vi "slow_control_alpha_07.vi"() -> ()   [LabVIEW 2018]
uses:
  <vilib>/DAQmx/read.llb/DAQmx Read (Analog 1D DBL NChan 1Samp).vi
  <vilib>/DAQmx/create/channels.llb/DAQmx Create Channel (AI-Voltage-Basic).vi
  <vilib>/DAQmx/miscellaneous.llb/DAQmx Fill In Error Info.vi
  <instrlib>/Lake Shore 335/Lake Shore 335.lvlib
  <instrlib>/CAEN PSM/CAEN PSM.lvlib
panel:
  out "Coldhead":dbl
  out "Heater":dbl
  out "Cycle number":i32
  out "TOBA tester":dbl[][](array[numeric])
  in  "Cycles to execute":dbl=5.0 format="%#_13g"
  out "Moving average Det. P":dbl
  in  "N samples":i32=20
  in  "Allows tabs on \nfront panel":T1(tab)
  in  "Heater range":u16(ring) items=["Off", "Low (On)", "Medium", "High"]
  in  "Setpoint (°C)":dbl=-100.0 format="%.1f"
  in  "PID settings":cluster{"P":dbl, "I":dbl, "D":dbl}={"P"=50.0, "I"=20.0, "D"=120.0}
  in  "COM-port LakeShore":refnum<visa-resource-name>
  in  "ID Query":bool=TRUE
  in  "COM-port CAEN 1":refnum<visa-resource-name>
  in  "COM-port CAEN 2":refnum<visa-resource-name>
  in  "Sensor 2 Offset":dbl=1.0 format="%#_13g"
  in  "Sensor 2 Mult. Factor":dbl=25.0 format="%#_13g"
  in  "Sensor 1 Offset":dbl=0.44736 format="%#_13g"
  in  "Sensor 1 Mult. Factor":dbl=25.0 format="%#_13g"
  in  "Sensor 3 Offset":dbl=1.0 format="%#_13g"
  in  "Sensor 3 Mult. Factor":dbl=50.0 format="%#_13g"
  in  "Sensor 4 Offset":dbl=1.0 format="%#_13g"
  in  "Sensor 4 Mult. Factor":dbl=10.0 format="%#_13g"
  out "Heater power (%) 2":cluster{timestamp[], dbl[]}[](graph)
  out "Temp B":dbl
  out "Temp A":dbl
  out "LakeShore readings 2":dbl[](array[numeric])
  in  "Detector Pressure":tag="cDAQ2Mod1/ai0"
  in  "Low Pressure":tag="cDAQ2Mod1/ai1"
  in  "High Pressure":tag="cDAQ2Mod1/ai2"
  in  "Flow Meter":tag="cDAQ2Mod1/ai3"
  out "Corrected P (3x bar, 1x SLPM)":dbl[](array[numeric])
  out "Raw P (Volt)":dbl[](array[numeric]) format="%0.4f"
  in  "Ignore Initialization Errors":bool caption="Ignore init. errors?"
  out "LakeShore status":bool
  out "NI mod1 (P) status":bool
  out "CAEN 1 status":bool
  out "CAEN 2 status":bool
  out "Initialization status":bool
  out "Heater power (%)":cluster{timestamp[], dbl[]}[](graph)
  out "Flow (SLPM)":cluster{timestamp[], dbl[]}[](graph)
  out "Pressure":cluster{timestamp[], dbl[]}[](graph)
  out "Phase Diagram":cluster{"X":dbl, "Y":dbl}[](graph)
  in  "Temp. Channel selector":string(combo)="Average 15 to 20"
  out "Temperature":cluster{timestamp[], dbl[]}[](graph)
  in  "N samples":i32=30
  out "Average Flow (SLPM)":dbl caption="Average Flow (SLPM), of"
  in  "Pause?":bool
  out "Integrated Flow (SL)":dbl
  in  "Reset?":bool
  out "LakeShore readings":dbl[](array[numeric])
  out "Temp. 1":dbl
  out "Temp. 2":dbl
  out "Temp. 3":dbl
  out "Temp. 4":dbl
  out "Temp. 5":dbl
  out "Temp. 6":dbl
  out "Temp. 7":dbl
  out "Temp. 8":dbl
  out "Temp. 9":dbl
  out "Temp. 10":dbl
  out "Temp. 11":dbl
  out "Temp. 12":dbl
  out "Temp. 13":dbl
  out "Temp. 14":dbl
  out "Temp. 15":dbl
  out "Temp. 16":dbl
  out "Temp. 17":dbl
  out "Temp. 18":dbl
  out "Temp. 19":dbl
  out "Temp. 20":dbl
  out "1 to 4":dbl[](array[numeric])
  out "5 to 8":dbl[](array[numeric])
  out "9 to 12":dbl[](array[numeric])
  out "13 to 16":dbl[](array[numeric])
  out "17 to 20":dbl[](array[numeric])
  in  "Temperature Channel selector":string(combo)="Average 15 to 20"
  out "Historical Large Phase Diagram":cluster{dbl[], dbl[]}[](graph)
  out "Large Phase Diagram":cluster{"X":dbl, "Y":dbl}[](graph)
  in  "Temperature Channel selector":string(combo)="Average 15 to 20"
  in  "Set to zero":bool
  out "Bottom gate":dbl(knob) scale=0.0..-3000.0
  out "Top gate":dbl(knob) scale=0.0..3000.0
  in  "Apply Voltage":bool
  in  "VSet (V)":dbl[](array[numeric])
  in  "IMax (uA)":dbl[](array[numeric])
  in  "VMax (V)":dbl[](array[numeric])
  out "Cathode":dbl(knob) scale=0.0..-5000.0
  out "Anode":dbl(knob) scale=0.0..4000.0
  out "PMT 2":dbl(knob) scale=0.0..1000.0
  out "PMT 1":dbl(knob) scale=1.0..1000.0
  out "Vmon (V)":dbl[](array[numeric])
  out "IMon (uA)":dbl[](array[numeric])
  in  "Read V every N cycles":i16=120
  in  "Reset anode":bool
  in  "Kill every Y minutes":i32=10
  in  "Keep off for X seconds":i32=10
  out "?":bool
  out "Killed":bool
  out "Restarted":bool
  out "Anode times":dbl[](array[numeric]) format="%_12f"
  out "Anode times 2":timestamp[](array[timestamp])
  in  "Kill voltage":bool
  in  "stop":bool
  out "Voltages":dbl[](array[numeric])
  out "Started up?":bool
  out "TOBA appended":dbl[][](array[numeric])
  in  "Read T every N cycles":i32=2
  out "Time until next cycle":dbl format="%.3g"
  in  "Time per cycle (s)":i32=2 caption="Time Target (s)"
  # "<- Proof of concept for New/Old T + New P"
  # "PMT 1"
  # "PMT 2"
  # "Anode"
  # "Cathode"
  # "Top gate"
  # "Bottom gate"
  # "Connection settings"
  # "Lakeshore settings"
  # "Pressure sensor settings"
  # "Gain (P) (XX.X)"
  # "Reset (I) (XX.X)"
  # "Rate (D) (X.X%)"
  # "Might need to split up NI-box com port.\nPreferable to task it with measuring T\nand P seperately.\nPerhaps need to set task per single channel."
  # "Heater tests"
  # "Move to Quick Temp tab ^"
  # "Alarm indicators"
  # "CAEN 1"
  # "Data"
  # "PMT 1"
  # "PMT 1"
  # "PMT 2"
  # "PMT 2"
  # "Anode"
  # "Anode"
  # "Cathode"
  # "Cathode"
  # "Top gate"
  # "Top gate"
  # "Bottom gate"
  # "Bottom gate"
  # "Settings"
  # "PMT 1"
  # "PMT 1"
  # "PMT 2"
  # "PMT 2"
  # "Anode"
  # "Anode"
  # "Cathode"
  # "Cathode"
  # "Top gate"
  # "Top gate"
  # "Bottom gate"
  # "Bottom gate"
  # "CAEN 2"
  # "PMT 1"
  # "PMT 2"
  # "Anode"
  # "Cathode"
  # "Needle gauges or other displays go here"
  # "Top gate"
  # "Bottom gate"
  # "Time of last reset"
  # "Time of last reactivation"
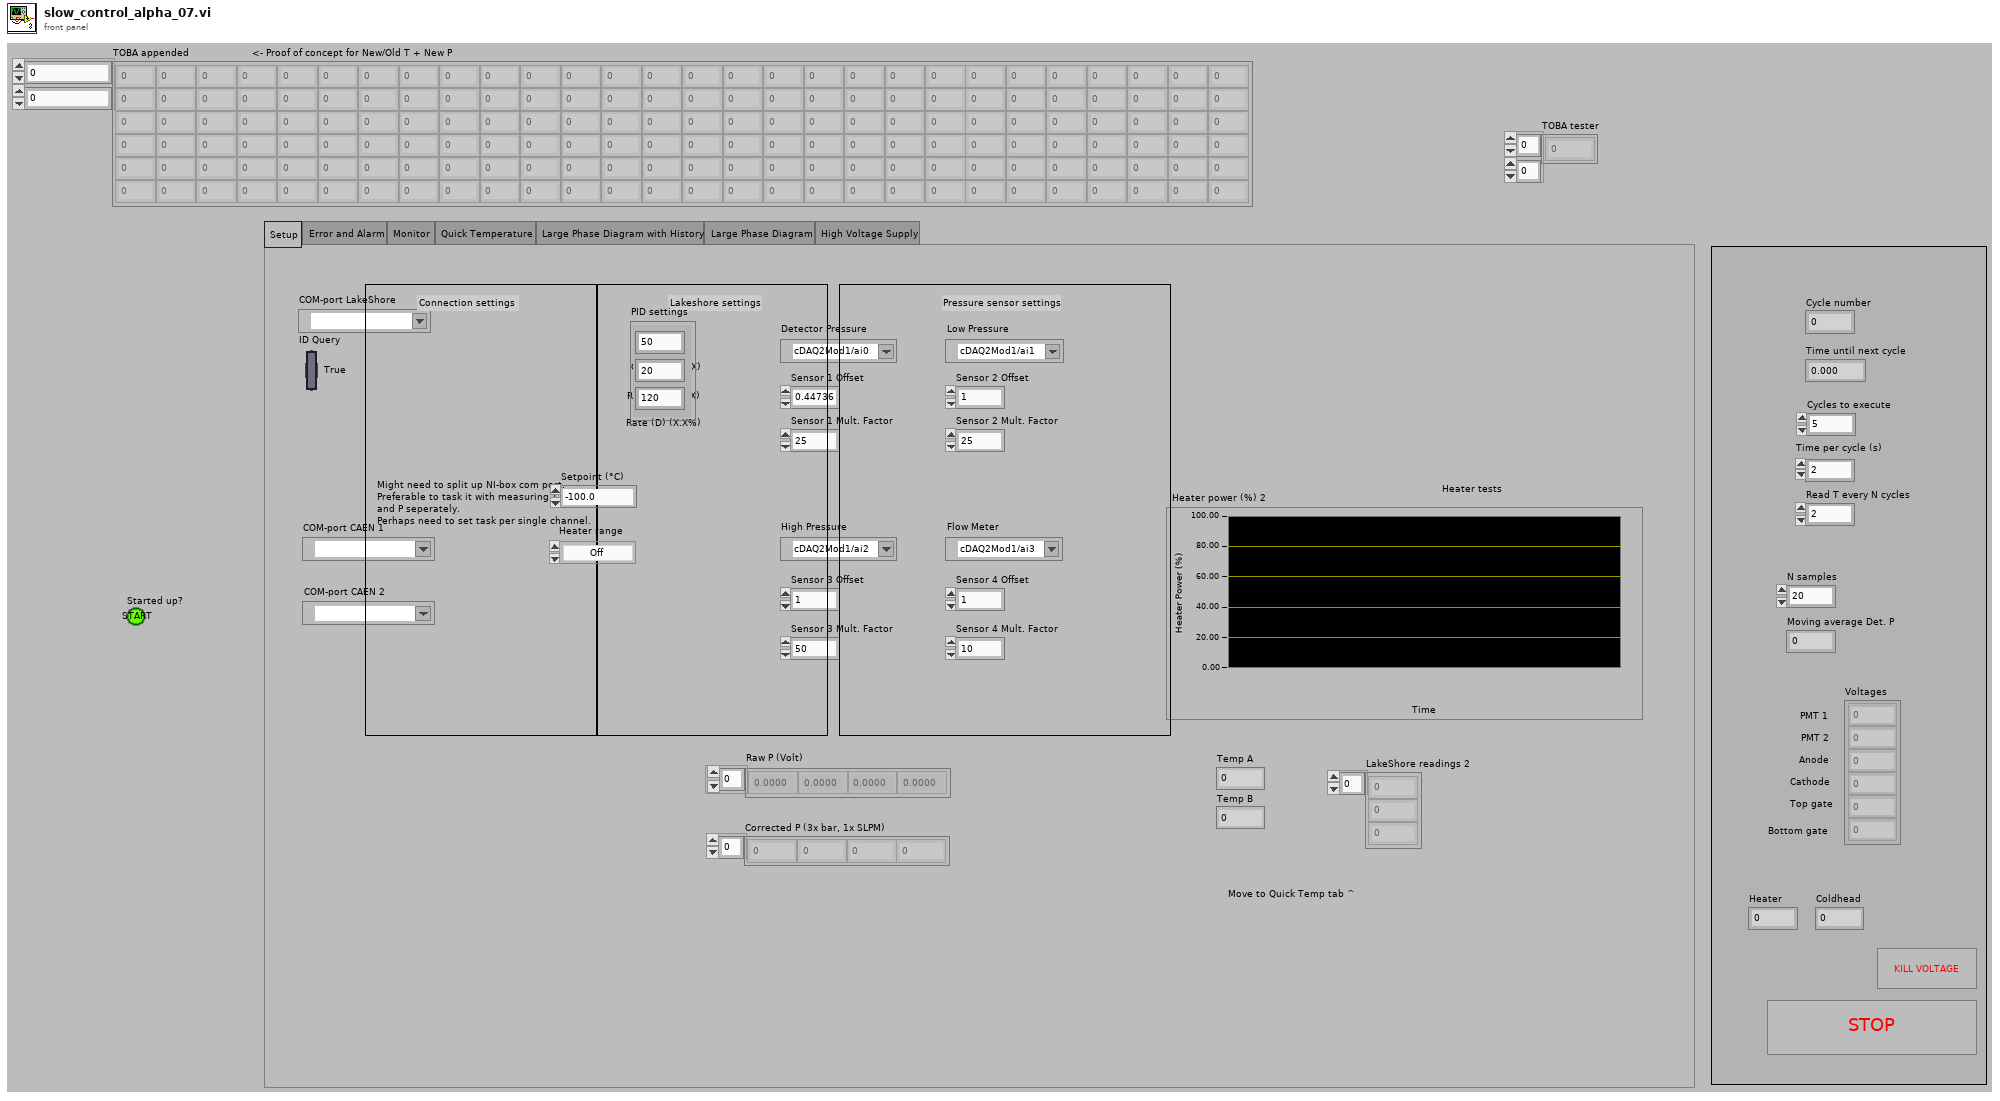
[diagram p1: front panel]
types:
  T1 = enum32{"Setup", "Error and Alarm", "Monitor", "Quick Temperature", "Large Phase Diagram with History", "Large Phase Diagram", "High Voltage Supply"}
  T2 = cluster{"Baud Rate":u32, "Parity":u16, "Data Bits":u16, "Stop Bits":u16, "Flow Control":u16}
  T3 = cluster{"VISA resource name out":refnum<visa-resource-name>, "error out":errorcluster}
  T4 = cluster{"task out":refnum<k21>, "error out":errorcluster}
  T5 = cluster{"Heater 1 (%)":dbl, "Heater 1 (%)":dbl}[]
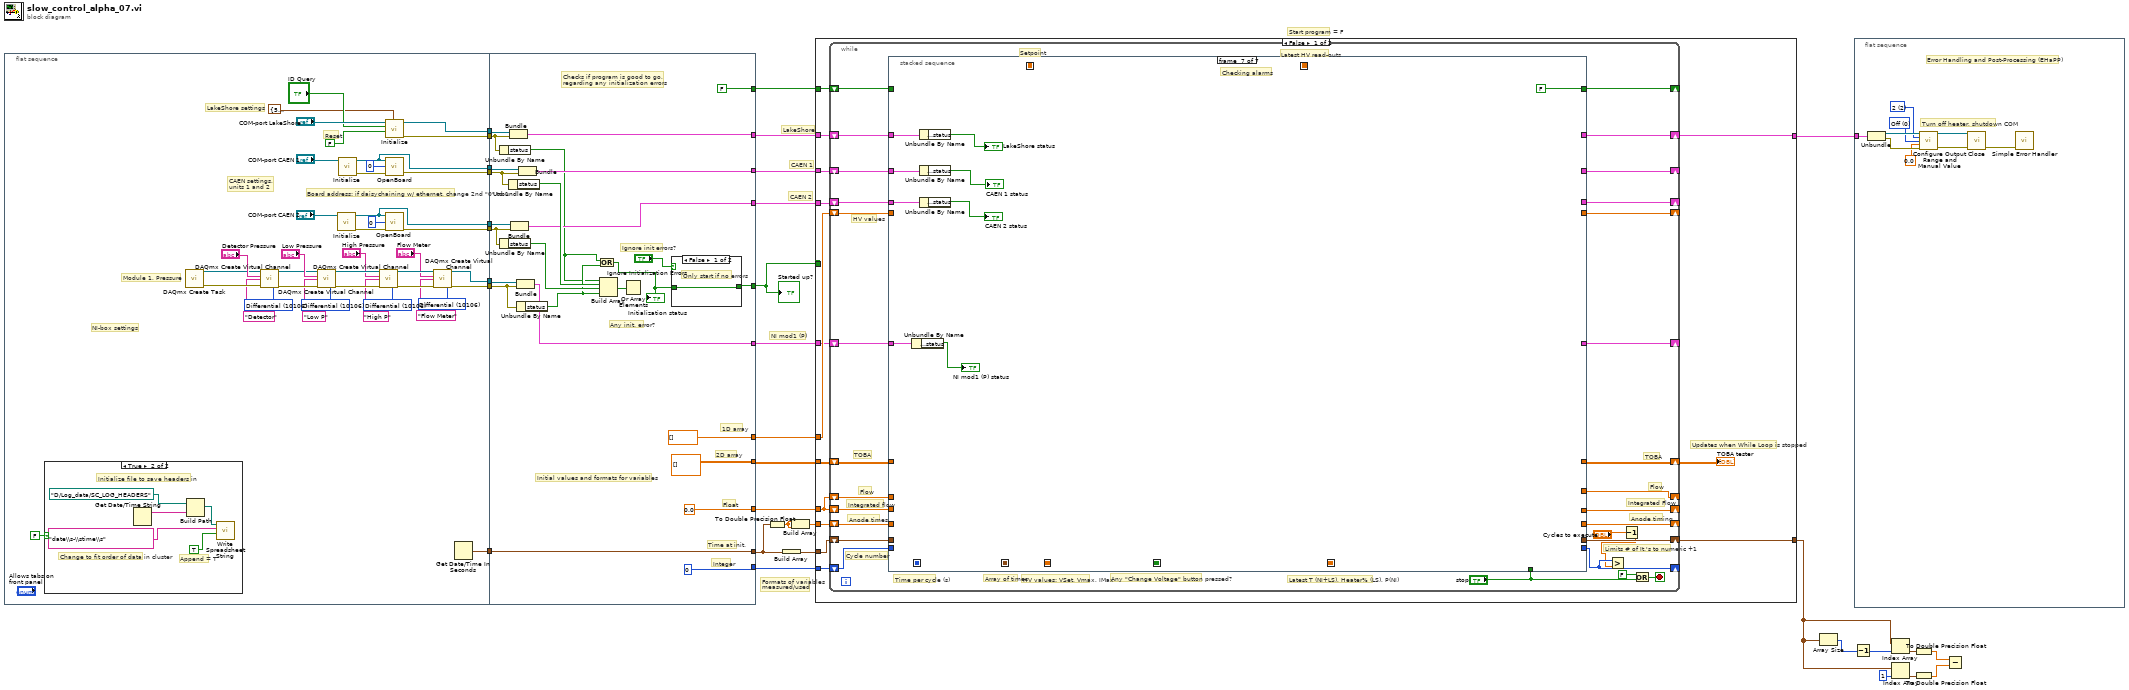
[diagram p0: block diagram]
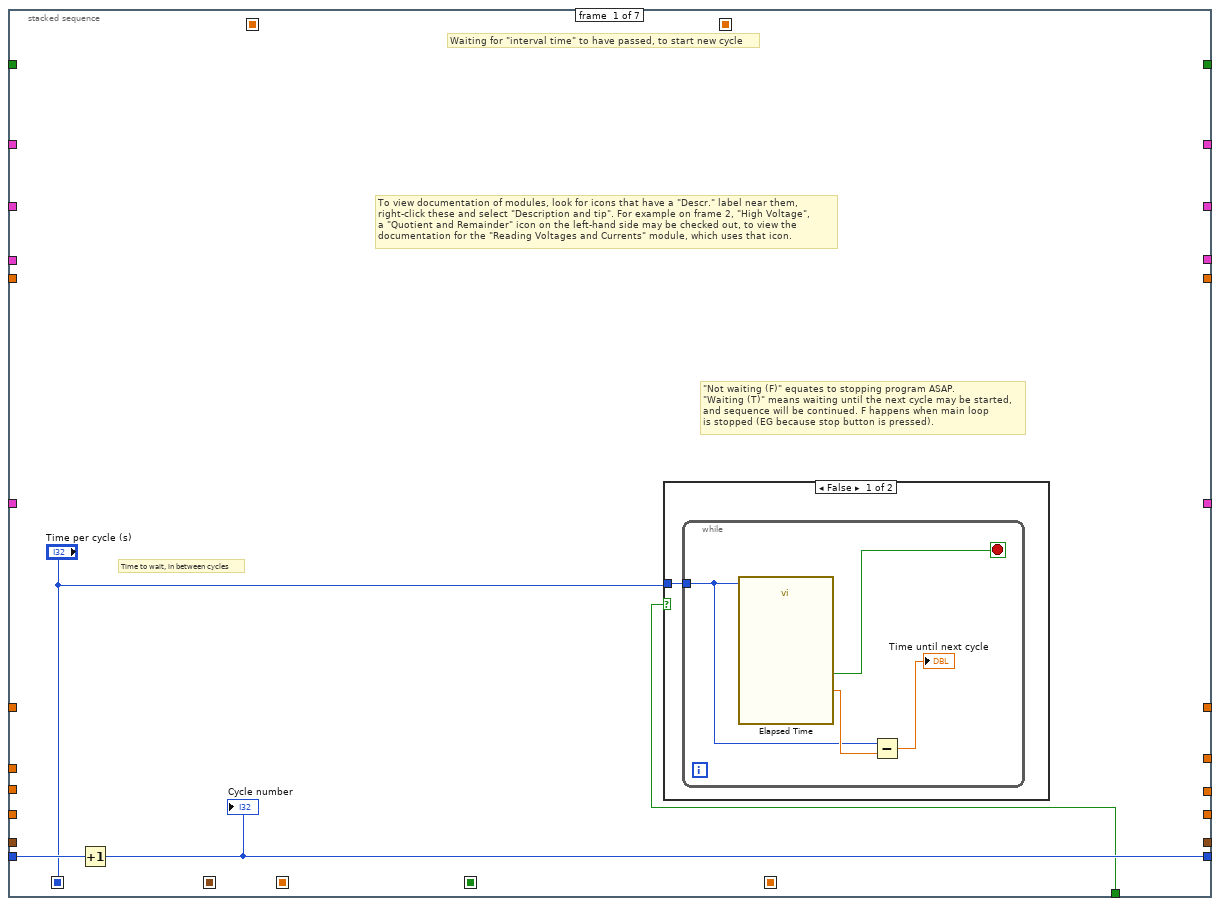
[diagram p2: hidden frame]
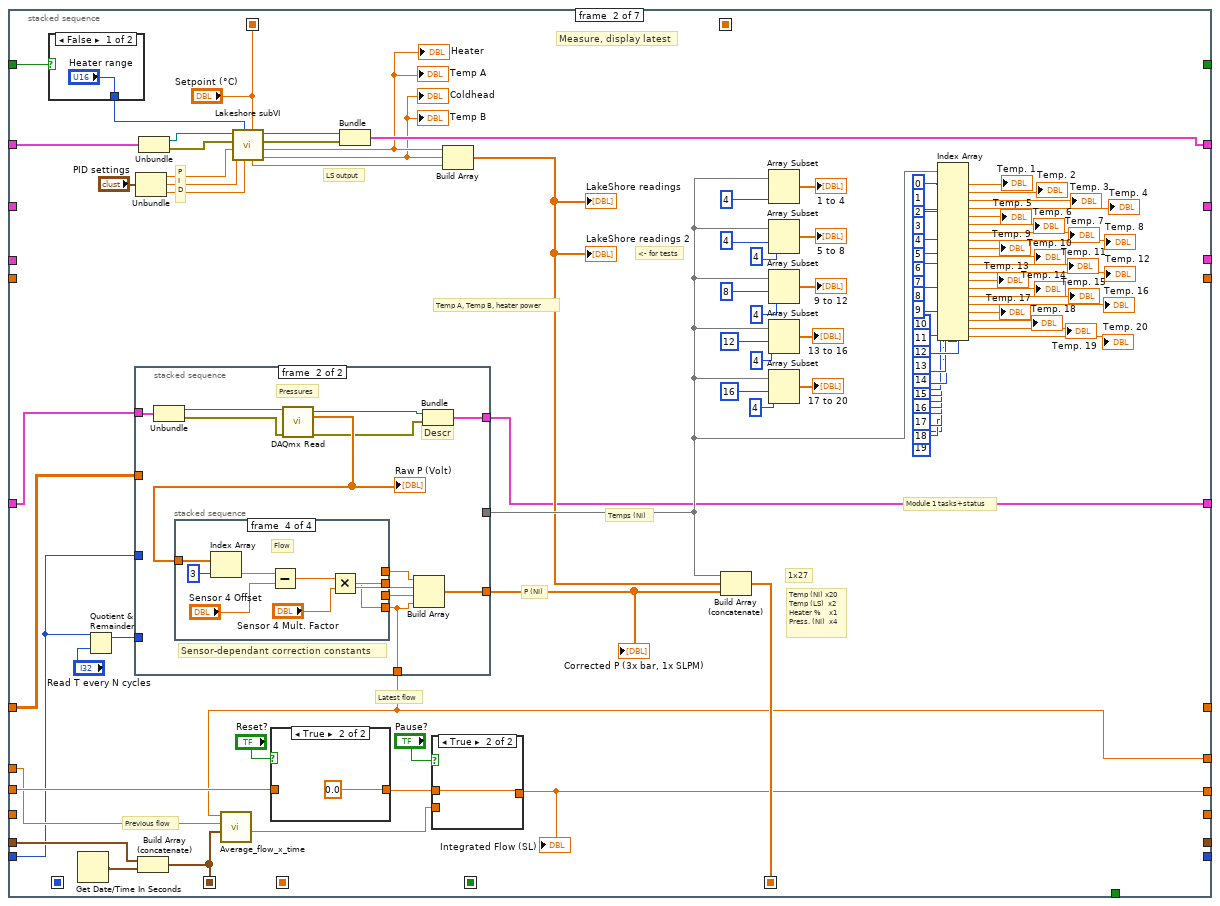
[diagram p4: hidden frame]
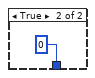
[diagram p5: hidden frame]
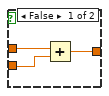
[diagram p7: hidden frame]
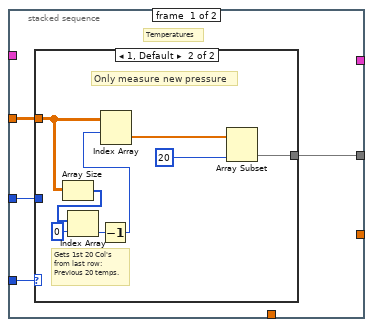
[diagram p8: hidden frame]
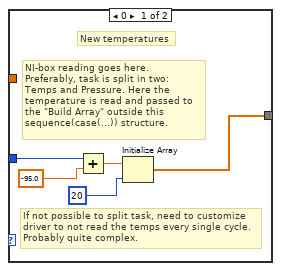
[diagram p9: hidden frame]
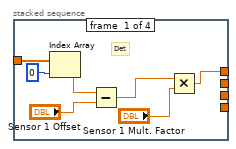
[diagram p10: hidden frame]
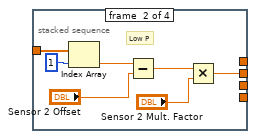
[diagram p11: hidden frame]
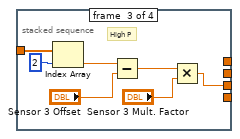
[diagram p12: hidden frame]
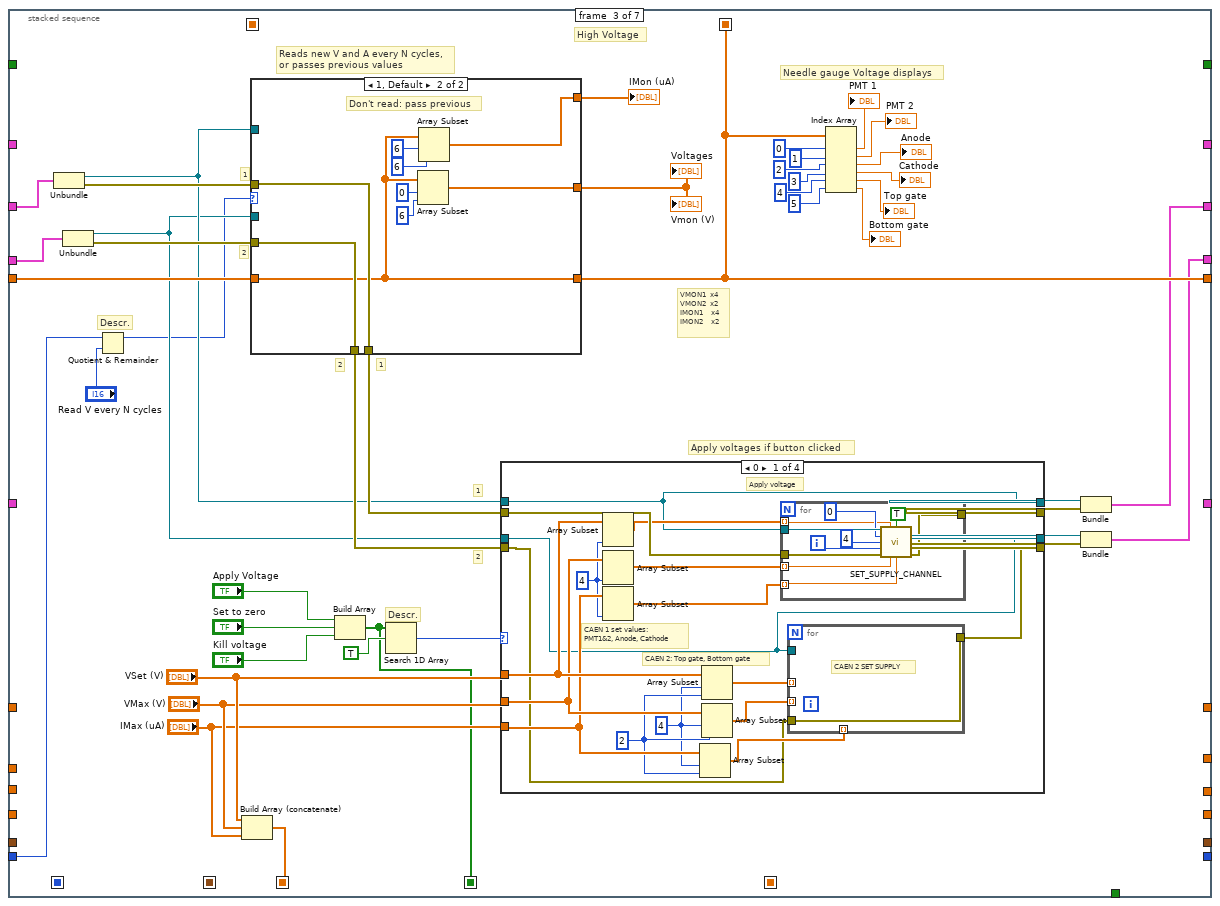
[diagram p13: hidden frame]
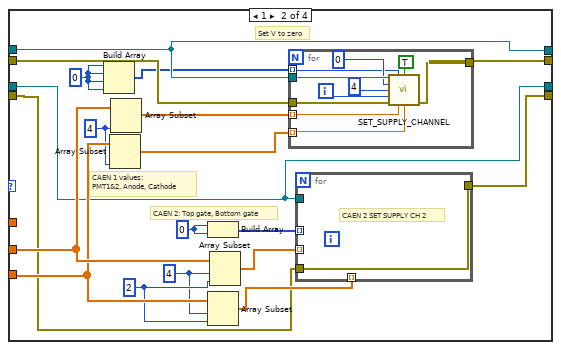
[diagram p14: hidden frame]
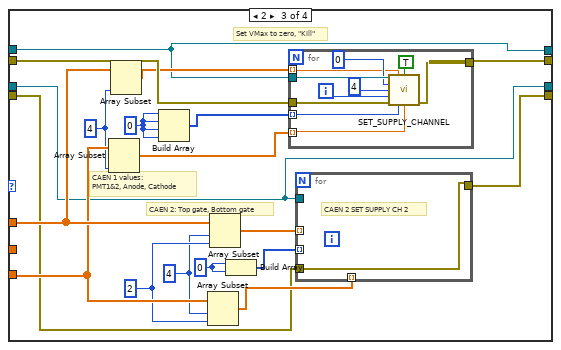
[diagram p15: hidden frame]
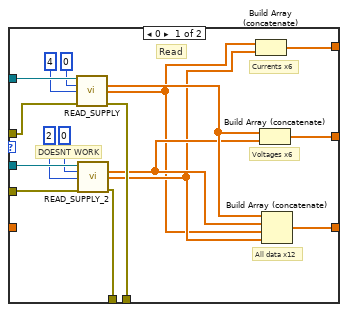
[diagram p17: hidden frame]
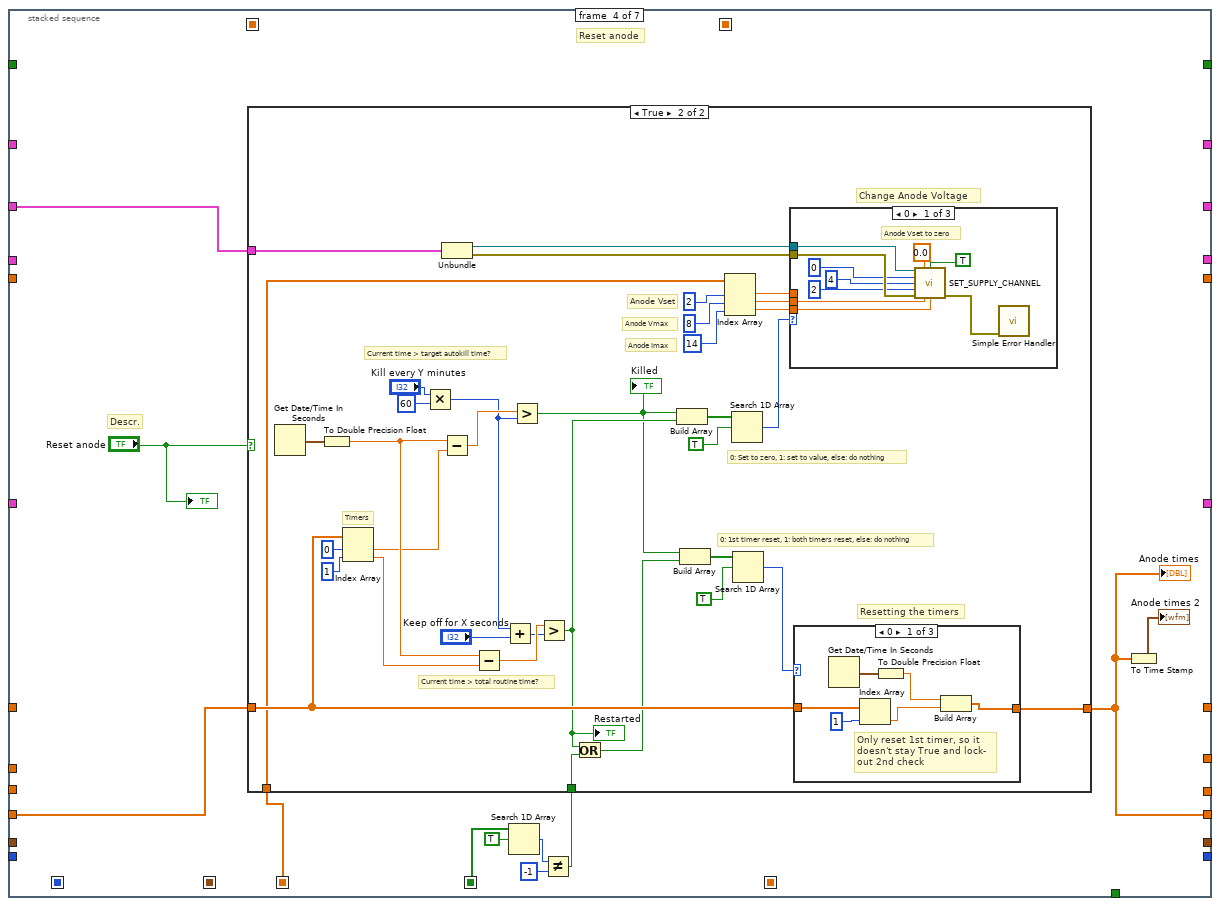
[diagram p18: hidden frame]
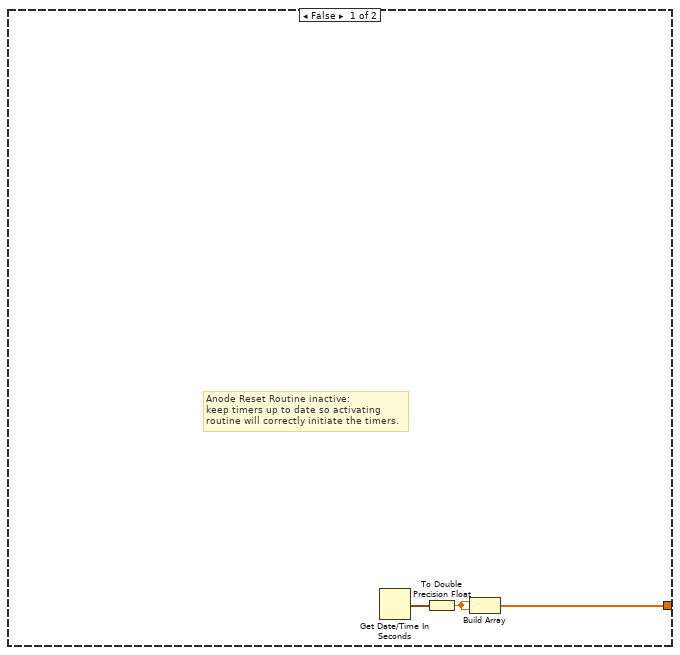
[diagram p19: hidden frame]
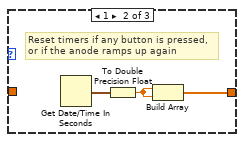
[diagram p20: hidden frame]
diagram:
  # "NI mod1 (P)"
  # "Start program = F"
  # "CAEN 2"
  # "CAEN 1"
  # "LakeShore"
  # "Formats of variables\nmeasured/used"
  n1 = flat-sequence {
    tunnel: [w69] -> w32
    tunnel: [w68] -> w31
    tunnel: [w55] -> w30
    tunnel: [w65] -> w29
    tunnel: [w34] -> w28
    tunnel: [w64] -> w22
    tunnel: [w60] -> w12
    tunnel: [w59] -> w11
    tunnel: [w33] -> w2
    tunnel: w32 -> [w100]
    tunnel: w31 -> [w99]
    tunnel: w30 -> [w97]
    tunnel: w29 -> [w96]
    tunnel: w28 -> [w86]
    tunnel: [w101] -> w9
    tunnel: [0.0] -> w8
    tunnel: [dbl[] []] -> w27
    tunnel: [dbl[][] []] -> w25
    tunnel: [0] -> w26
    tunnel: [w98] -> w24
    tunnel: [w95] -> w23
    tunnel: [w94] -> w7
    tunnel: w22 -> [w94]
    tunnel: w12 -> [w92]
    tunnel: w11 -> [w91]
    tunnel: [w90] -> w10
    tunnel: [FALSE] -> w3
    tunnel: w2 -> [w87]
    tunnel: [w85] -> w1
    frame #0 {
      w36 = 10106 items=["Default"=-1, "RSE"=10083, "NRSE"=10078, "Differential"=10106, "Pseudodifferential"=12529] ("input terminal configuration")
      w40 = 10106 items=["Default"=-1, "RSE"=10083, "NRSE"=10078, "Differential"=10106, "Pseudodifferential"=12529] ("input terminal configuration")
      w49 = 10106 items=["Default"=-1, "RSE"=10083, "NRSE"=10078, "Differential"=10106, "Pseudodifferential"=12529] ("input terminal configuration")
      w52 = 10106 items=["Default"=-1, "RSE"=10083, "NRSE"=10078, "Differential"=10106, "Pseudodifferential"=12529] ("input terminal configuration")
      # "Module 1, Pressure"
      # "Board address: if daisychaining w/ ethernet, change 2nd \"0\" to 1"
      # "NI-box settings"
      # "CAEN settings,\nunits 1 and 2"
      # "Reset"
      # "LakeShore settings"
      n2 = case shown="True" FALSE {
        frame False {
        }
        frame True {
          # "Append = T"
          # "Change to fit order of data in cluster"
          # "Initialize file to save headers in"
          n3 = Get Date/Time String() -> (date string=w77:string)  [unwired: 3 in, 1 out]
          n4 = Build Path(base path=path "D:/Log_data/SC_LOG_HEADERS", name or relative path=w77) -> (appended path=w76:path)
          n5 = call <vilib>:"Write Spreadsheet String.vi"("append to file? (new file:F)"=TRUE, "spreadsheet string"="date\\s-\\stime\\s", "file path (dialog if empty)"=w76) -> ()  [unwired: 7 in, 2 out]
        }
      }
      n6 = call <vilib>:"DAQmx Create Task.vi"() -> ("task out"=w51:refnum<k21>, "error out"=w53:errorcluster)  [unwired: 14 in]
      n7 = call-poly <vilib>:"DAQmx Create Virtual Channel.vi"("task in"=w51, "input terminal configuration"=w52, "physical channels"="Detector Pressure", "name to assign"="Detector", "error in"=w53) -> ("task out"=w47:refnum<k21>, "error out"=w48:errorcluster)  [unwired: 9 in]
      n8 = call-poly <vilib>:"DAQmx Create Virtual Channel.vi"("task in"=w47, "input terminal configuration"=w49, "physical channels"="Low Pressure", "name to assign"="Low P", "error in"=w48) -> ("task out"=w44:refnum<k21>, "error out"=w42:errorcluster)  [unwired: 9 in]
      n9 = call <instrlib>:"Initialize.vi"("VISA resource name"="COM-port CAEN 2") -> ("error out"=w61:errorcluster, "VISA resource name out"=w60:refnum<visa-resource-name>)  [unwired: 9 in]
      n10 = call <instrlib>:"Initialize.vi"("VISA resource name"="COM-port CAEN 1") -> ("error out"=w66:errorcluster, "VISA resource name out"=w55:refnum<visa-resource-name>)  [unwired: 9 in]
      n11 = call-poly <vilib>:"DAQmx Create Virtual Channel.vi"("task in"=w44, "input terminal configuration"=w40, "physical channels"="High Pressure", "name to assign"="High P", "error in"=w42) -> ("task out"=w39:refnum<k21>, "error out"=w38:errorcluster)  [unwired: 9 in]
      n12 = call <instrlib>:"OpenBoard.vi"("error in (no error)"=w61, "Board Address"=u8 0, "VISA resource name"=w60) -> ("error out"=w59:errorcluster)  [unwired: 7 in, 1 out]
      n13 = call <instrlib>:"Initialize.vi"("Serial Configuration"=T2 {"Baud Rate"=57600, "Parity"=1, "Data Bits"=7, "Stop Bits"=10, "Flow Control"=0}, "Reset (True)"=FALSE ("Reset (LakeShore)"), "ID Query (True)"="ID Query", "VISA resource name"="COM-port LakeShore") -> ("error out"=w68:errorcluster, "VISA resource name out"=w69:refnum<visa-resource-name>)  [unwired: 6 in]
      n14 = call <instrlib>:"OpenBoard.vi"("error in (no error)"=w66, "Board Address"=0, "VISA resource name"=w55) -> ("error out"=w65:errorcluster)  [unwired: 7 in, 1 out]
      n15 = call-poly <vilib>:"DAQmx Create Virtual Channel.vi"("task in"=w39, "input terminal configuration"=w36, "physical channels"="Flow Meter", "name to assign"="Flow Meter", "error in"=w38) -> ("task out"=w33:refnum<k21>, "error out"=w34:errorcluster)  [unwired: 9 in]
      n16 = Get Date/Time In Seconds() -> (seconds since 1Jan1904=w64:timestamp)
    }
    frame #1 {
      # "Initial values and formats for variables"
      # "Time at init."
      # "Integer"
      # "2D array"
      # "1D array"
      # "Float"
      # "Checks if program is good to go,\nregarding any initialization errors"
      # "Ignore init errors?"
      # "Any init. error?"
      n17 = Unbundle By Name(w99) -> ("status"=w79:bool)
      n18 = Unbundle By Name(w91) -> ("status"=w93:bool)
      n19 = Unbundle By Name(w96) -> ("status"=w102:bool)
      n20 = Bundle("VISA resource name out"=w100, "error out"=w99) -> (w98:T3)  [unwired: 1 in]
      n21 = Bundle("VISA resource name out"=w92, "error out"=w91) -> (w90:T3)  [unwired: 1 in]
      n22 = Unbundle By Name(w86) -> ("status"=w80:bool)
      n23 = Bundle("task out"=w87, "error out"=w86) -> (w85:T4)  [unwired: 1 in]
      n24 = Bundle("VISA resource name out"=w97, "error out"=w96) -> (w95:T3)  [unwired: 1 in]
      n25 = Or(x=w79, y=w80) -> (x .or. y?=w78:bool)
      "Initialization status" <- w78
      n26 = Build Array(w79, w102, w80, w93) -> (w103:bool[])
      n27 = Or Array Elements(Boolean array=w103) -> ()  [unwired: 1 out]
      n28 = case shown="False" "Ignore Initialization Errors" {
        tunnel: [w104 FALSE] -> w101
        tunnel: w78 -> [w104 _]
        frame False {
          # "Only start if no errors"
        }
        frame True {
          # "Always start program"
        }
      }
    }
  }
  n29 = To Double Precision Float(number=w7) -> (double precision float=w6:dbl)
  n30 = Build Array(w7) -> (w21:timestamp[])
  n31 = Build Array(w6, w6) -> (w5:dbl[])
  n32 = case shown="False" w9 {
    selector: w9 -> [_ w721]
    tunnel: [_ w721] -> _
    tunnel: w27 -> [w112 _]
    tunnel: w26 -> [w119 _]
    tunnel: w25 -> [w118 _]
    tunnel: w24 -> [w113 w719]
    tunnel: w23 -> [w115 _]
    tunnel: w21 -> [w117 _]
    tunnel: [w116 timestamp[] []] -> w17
    tunnel: w10 -> [w114 _]
    tunnel: w8 -> [w107 _]
    tunnel: w5 -> [w111 _]
    tunnel: [w109 w719] -> w4
    tunnel: w3 -> [w108 _]
    tunnel: w1 -> [w106 _]
    frame False {
      # "Updates when While Loop is stopped"
      n33 = while {
        shift-right: [w143] -> _
        shift-left: w119 -> [w148]
        shift-right: [w145] -> w110
        shift-left: w118 -> [w134]
        shift-right: [w135] -> w116
        shift-left: w117 -> [w144]
        shift-right: [w137] -> _
        shift-left: w115 -> [w126]
        shift-right: [w139] -> _
        shift-left: w112 -> [w142]
        shift-right: [w136] -> _
        shift-left: w114 -> [w141]
        shift-right: [w138] -> w109
        shift-left: w113 -> [w140]
        shift-right: [w133] -> _
        shift-left: w107 -> [w128]
        shift-right: [w130] -> _
        shift-left: w107 -> [w129]
        shift-right: [w125] -> _
        shift-left: w111 -> [w127]
        shift-right: [w122] -> _
        shift-left: w108 -> [w123]
        shift-right: [w120] -> _
        shift-left: w106 -> [w121]
        stop <- w146 stop-if-true
        # "Any \"Change Voltage\" button pressed?"
        # "Setpoint"
        # "Anode timing"
        # "Anode times"
        # "Integrated flow"
        # "Flow"
        # "Flow"
        # "Integrated Flow"
        # "TOBA"
        # "Array of times"
        # "Latest HV read-outs"
        # "Time per cycle (s)"
        # "Cycle number"
        # "HV values: VSet, Vmax, IMax"
        # "HV values"
        # "TOBA"
        # "Latest T (NI+LS), Heater% (LS), P(NI)"
        # "Limits # of It.'s to numeric +1"
        n34 = stacked-sequence {
          seq-local: [_ w245 _ _ _ _ _] -> [_ _ _ _ w591 w709 _]
          seq-local: [_ _ w320 _ _ _ _] -> [_ _ _ w483 _ _ _]
          seq-local: ["Time per cycle (s)" _ _ _ _ _ _] -> [_ _ _ _ _ w705 _]
          seq-local: [_ _ w335 _ _ _ _] -> [_ _ _ _ _ w704 _]
          seq-local: [_ w170 _ _ _ _ _] -> [_ _ _ _ w571 _ _]
          seq-local: [_ _ w314 _ _ _ _] -> [_ _ _ w486 _ _ _]
          seq-local: [_ "Setpoint (°C)" _ _ _ _ _] -> [_ _ _ _ _ w708 _]
          tunnel: [w151 _ _ _ _ _ _] -> w143
          tunnel: "stop" -> [w150 _ _ _ _ _ _]
          tunnel: w148 -> [w152 w158 w349 _ _ _ _]
          tunnel: w134 -> [_ w246 _ _ w598 _ _]
          tunnel: [_ _ _ _ w555 _ _] -> w145
          tunnel: w144 -> [_ w233 _ _ _ _ _]
          tunnel: w126 -> [_ _ w356 w484 _ _ w716]
          tunnel: w142 -> [_ _ w354 _ _ _ _]
          tunnel: w141 -> [_ _ w353 _ _ _ w715]
          tunnel: w140 -> [_ w234 _ _ _ _ w713]
          tunnel: [_ w235 _ _ _ _ _] -> w138
          tunnel: [_ _ w335 _ _ _ _] -> w139
          tunnel: [_ _ w328 _ _ _ _] -> w137
          tunnel: [_ _ w325 _ _ _ _] -> w136
          tunnel: [_ _ _ _ w571 _ _] -> w135
          tunnel: w128 -> [_ w227 _ _ _ _ _]
          tunnel: [_ w228 _ _ _ _ _] -> w133
          tunnel: [_ w168 _ _ _ _ _] -> w130
          tunnel: w129 -> [_ w167 _ _ _ _ _]
          tunnel: w127 -> [_ _ _ w485 _ _ _]
          tunnel: [_ _ _ w479 _ _ _] -> w125
          tunnel: w123 -> [_ w162 _ _ _ _ _]
          tunnel: [_ _ _ _ _ _ FALSE] -> w122
          tunnel: w121 -> [_ w160 _ _ _ _ w711]
          tunnel: [_ w159 _ _ _ _ _] -> w120
          frame #0 {
            # "To view documentation of modules, look for icons that have a \"Descr.\" label near them,\nright-click these and select \"Description and tip\". For example on frame 2, \"High Voltage\",\na \"Quotient and Remainder\" icon on the left-hand side may be checked out, to view the\ndocumentation for the \"Reading Voltages and Currents\" module, which uses that icon."
            # "Time to wait, in between cycles"
            # "\"Not waiting (F)\" equates to stopping program ASAP.\n\"Waiting (T)\" means waiting until the next cycle may be started,\nand sequence will be continued. F happens when main loop \nis stopped (EG because stop button is pressed)."
            # "Waiting for \"interval time\" to have passed, to start new cycle"
            n35 = Increment(x=w152) -> (x+1=w151:i32)
            "Cycle number" <- w151
            n36 = case shown="False" w150 {
              tunnel: "Time per cycle (s)" -> [w153 _]
              frame False {
                n37 = while {
                  tunnel: w153 -> [w155]
                  stop <- w157 stop-if-true
                  n38 = call "Elapsed Time"("Time Target (s)"=w155) -> ("Elapsed Time (s)"=w156:dbl, "Time has Elapsed"=w157:bool)  [unwired: 11 in, 6 out]
                  n39 = Subtract(x=w155, y=w156) -> (x-y=→"Time until next cycle":dbl)
                }
              }
              frame True {
              }
            }
          }
          frame #1 {
            # "Previous flow"
            # "Latest flow"
            # "Module 1 tasks+status"
            # "<- for tests"
            # "P (NI)"
            # "Temps (NI)"
            # "1x27"
            # "LS output"
            # "Temp (NI) x20\nTemp (LS)  x2\nHeater %    x1\nPress. (NI)  x4"
            # "Temp A, Temp B, heater power"
            # "P\nI\nD"
            # "Measure, display latest"
            n40 = case shown="False" w162 {
              tunnel: ["Heater range" 0] -> w238
              frame False {
              }
              frame True {
              }
            }
            n41 = Get Date/Time In Seconds() -> (seconds since 1Jan1904=w232:timestamp)
            n42 = Quotient & Remainder(x=w158, y="Read T every N cycles") -> (x-y*floor(x/y)=w247:i32)  [unwired: 1 out]
            n43 = stacked-sequence {
              tunnel: w247 -> [w260 _]
              tunnel: [w259 _] -> w169
              tunnel: [_ w282] -> w231
              tunnel: w246 -> [w258 _]
              tunnel: w158 -> [w257 _]
              tunnel: [_ w281] -> w168
              tunnel: w160 -> [_ w280]
              tunnel: [_ w274] -> w159
              frame #0 {
                # "Temperatures"
                n44 = case shown="1, Default" w260 {
                  tunnel: w258 -> [_ w270]
                  tunnel: [w263 w266] -> w259
                  tunnel: w257 -> [w262 _]
                  frame 0 {
                    # "If not possible to split task, need to customize\ndriver to not read the temps every single cycle.\nProbably quite complex."
                    # "NI-box reading goes here.\nPreferably, task is split in two: \nTemps and Pressure. Here the \ntemperature is read and passed to \nthe \"Build Array\" outside this \nsequence(case(...)) structure."
                    # "New temperatures"
                    n45 = Add(x=w262, y=-95.0 ("element")) -> (x+y=w265:dbl)
                    n46 = Initialize Array(w265, 20) -> (w263:dbl[])
                  }
                  frame 1, Default {
                    # "Gets 1st 20 Col's\nfrom last row:\nPrevious 20 temps."
                    # "Only measure new pressure"
                    n47 = Array Size(array=w270) -> (size(s)=w272:i32[])
                    n48 = Index Array(array=w272, index=0) -> (element=w273:i32)
                    n49 = Decrement(x=w273) -> (x-1=w269:i32)
                    n50 = Index Array(array=w270, index (row)=w269) -> (element=w268:dbl[])  [unwired: 1 in]
                    n51 = Array Subset(array=w268, length=20) -> (w266:dbl[])  [unwired: 1 in]
                  }
                }
              }
              frame #1 {
                # "Descr"
                # "Sensor-dependant correction constants"
                # "Pressures"
                n52 = Unbundle(w280) -> ("task out"=w279:refnum<k21>, "error out"=w278:errorcluster)
                n53 = call-poly <vilib>:"DAQmx Read.vi"("task/channels in"=w279, "error in"=w278) -> ("task out"=w276:refnum<k21>, "data"=w277:dbl[], "error out"=w275:errorcluster)  [unwired: 11 in]
                "Raw P (Volt)" <- w277
                n54 = stacked-sequence {
                  tunnel: w277 -> [w287 w299 w306 w313]
                  tunnel: [w288 _ _ _] -> w285
                  tunnel: [_ w294 _ _] -> w284
                  tunnel: [_ _ w301 _] -> w283
                  tunnel: [_ _ _ w309] -> w281
                  frame #0 {
                    # "Det"
                    n55 = Index Array(array=w287, index=0) -> (element=w286:dbl)
                    n56 = Subtract(x=w286, y="Sensor 1 Offset") -> (x-y=w290:dbl)
                    n57 = Multiply(x=w290, y="Sensor 1 Mult. Factor") -> (x*y=w288:dbl)
                  }
                  frame #1 {
                    # "Low P"
                    n58 = Index Array(array=w299, index=1) -> (element=w293:dbl)
                    n59 = Subtract(x=w293, y="Sensor 2 Offset") -> (x-y=w296:dbl)
                    n60 = Multiply(x=w296, y="Sensor 2 Mult. Factor") -> (x*y=w294:dbl)
                  }
                  frame #2 {
                    # "High P"
                    n61 = Index Array(array=w306, index=2) -> (element=w300:dbl)
                    n62 = Subtract(x=w300, y="Sensor 3 Offset") -> (x-y=w303:dbl)
                    n63 = Multiply(x=w303, y="Sensor 3 Mult. Factor") -> (x*y=w301:dbl)
                  }
                  frame #3 {
                    # "Flow"
                    n64 = Index Array(array=w313, index=3) -> (element=w308:dbl)
                    n65 = Subtract(x=w308, y="Sensor 4 Offset") -> (x-y=w311:dbl)
                    n66 = Multiply(x=w311, y="Sensor 4 Mult. Factor") -> (x*y=w309:dbl)
                  }
                }
                n67 = Build Array(w285, w284, w283, w281) -> (w282:dbl[])
                n68 = Bundle("task out"=w276, "error out"=w275) -> (w274:T4)  [unwired: 1 in]
              }
            }
            "Corrected P (3x bar, 1x SLPM)" <- w231
            n69 = Unbundle("PID settings") -> ("P"=w241:dbl, "I"=w240:dbl, "D"=w239:dbl)
            n70 = Build Array (concatenate)(w233, w232) -> (w170:timestamp[])
            n71 = Unbundle(w234) -> ("VISA resource name out"=w243:refnum<visa-resource-name>, "error out"=w242:errorcluster)
            n72 = call "Average_flow_x_time.vi"("Array of timestamps"=w170, "Previous Flow"=w167, "Latest Flow"=w168) -> ("Volume (SL)"=w226:dbl)  [unwired: 8 in]
            n73 = call "Lakeshore subVI.vi"("Setpoint"="Setpoint (°C)", "Rate (D) (X.X %)"=w239, "Range"=w238, "Reset (I) (XX.X)"=w240, "Gain (P) (XX.X)"=w241, "error in (no error)"=w242, "VISA resource name"=w243) -> ("Input B"=w165:dbl, "Input A"=w166:dbl, "error out"=w236:errorcluster, "VISA resource name out"=w237:refnum<visa-resource-name>, "Heater 1 (%)"=w164:dbl)
            "Temp A" <- w166
            "Temp B" <- w165
            "Coldhead" <- w165
            "Heater" <- w166
            n74 = case shown="True" "Reset?" {
              tunnel: w227 -> [w251 _]
              tunnel: [w251 0.0] -> w225
              frame False {
              }
              frame True {
              }
            }
            n75 = Bundle("VISA resource name out"=w237, "error out"=w236) -> (w235:T3)  [unwired: 1 in]
            n76 = case shown="True" "Pause?" {
              tunnel: w226 -> [w255 _]
              tunnel: w225 -> [w254 w256]
              tunnel: [w253 w256] -> w228
              frame False {
                n77 = Add(x=w254, y=w255) -> (x+y=w253:dbl)
              }
              frame True {
              }
            }
            "Integrated Flow (SL)" <- w228
            n78 = Build Array(w166, w165, w164) -> (w163:dbl[])
            "LakeShore readings" <- w163
            "LakeShore readings 2" <- w163
            n79 = Build Array (concatenate)(w169, w163, w231) -> (w245:dbl[])
            n80 = Array Subset(array=w169, length=4) -> (→"1 to 4":dbl[])  [unwired: 1 in]
            n81 = Array Subset(array=w169, index=4, length=4 ("index")) -> (→"5 to 8":dbl[])
            n82 = Array Subset(array=w169, index=8, length=4 ("index")) -> (→"9 to 12":dbl[])
            n83 = Array Subset(array=w169, index=12, length=4 ("index")) -> (→"13 to 16":dbl[])
            n84 = Array Subset(array=w169, index=16, length=4 ("index")) -> (→"17 to 20":dbl[])
            n85 = Index Array(array=w169, index #1=0, index #2=1, index #3=2, index #4=3, index #5=4, index #6=5, index #7=6, index #8=7, index #9=8, index #10=9, index #11=10, index #12=11, index #13=12, index #14=13, index #15=14, index #16=15, index #17=16, index #18=17, index #19=18, index #20=19) -> (element #1=→"Temp. 1":dbl, element #2=→"Temp. 2":dbl, element #3=→"Temp. 3":dbl, element #4=→"Temp. 4":dbl, element #5=→"Temp. 5":dbl, element #6=→"Temp. 6":dbl, element #7=→"Temp. 7":dbl, element #8=→"Temp. 8":dbl, element #9=→"Temp. 9":dbl, element #10=→"Temp. 10":dbl, element #11=→"Temp. 11":dbl, element #12=→"Temp. 12":dbl, element #13=→"Temp. 13":dbl, element #14=→"Temp. 14":dbl, element #15=→"Temp. 15":dbl, element #16=→"Temp. 16":dbl, element #17=→"Temp. 17":dbl, element #18=→"Temp. 18":dbl, element #19=→"Temp. 19":dbl, element #20=→"Temp. 20":dbl)
          }
          frame #2 {
            # "Apply voltages if button clicked"
            # "2"
            # "1"
            # "Descr."
            # "Descr."
            # "VMON1  x4 \nVMON2  x2\nIMON1    x4\nIMON2    x2"
            # "Needle gauge Voltage displays"
            # "1"
            # "2"
            # "1"
            # "2"
            # "Reads new V and A every N cycles,\nor passes previous values"
            # "High Voltage"
            n86 = Unbundle(w356) -> ("VISA resource name out"=w331:refnum<visa-resource-name>, "error out"=w355:errorcluster)
            n87 = Unbundle(w353) -> ("VISA resource name out"=w330:refnum<visa-resource-name>, "error out"=w352:errorcluster)
            n88 = Quotient & Remainder(x=w349, y="Read V every N cycles") -> (x-y*floor(x/y)=w315:i32)  [unwired: 1 out]
            n89 = Build Array (concatenate)("VSet (V)", "VMax (V)", "IMax (uA)") -> (w320:dbl[])
            n90 = case shown="1, Default" w315 {
              tunnel: w331 -> [w466 _]
              tunnel: w355 -> [w465 w474]
              tunnel: w354 -> [_ w470]
              tunnel: w330 -> [w460 _]
              tunnel: w352 -> [w459 w475]
              tunnel: [w456 w475] -> w332
              tunnel: [w462 w474] -> w333
              tunnel: [w461 w470] -> w335
              tunnel: [w453 w471] -> w351
              tunnel: [w450 w467] -> w350
              frame 0 {
                # "DOESNT WORK"
                # "All data x12"
                # "Voltages x6"
                # "Currents x6"
                # "Read"
                n91 = call "READ_SUPPLY.vi"("VISA resource name"=w466, "Board address"=u8 0, "NChannels"=u8 4, "error in (no error)"=w465) -> ("VMon values (V)"=w455:dbl[], "IMon values (uA)"=w451:dbl[], "error out"=w462:errorcluster)  [unwired: 9 in]
                n92 = call "READ_SUPPLY_2.vi"("VISA resource name"=w460, "Board address"=u8 0, "NChannels"=u8 2, "error in (no error)"=w459) -> ("VMon values (V)"=w454:dbl[], "IMon values (uA)"=w452:dbl[], "error out"=w456:errorcluster)  [unwired: 9 in]
                n93 = Build Array (concatenate)(w451, w452) -> (w450:dbl[])
                n94 = Build Array (concatenate)(w455, w454) -> (w453:dbl[])
                n95 = Build Array (concatenate)(w455, w454, w451, w452) -> (w461:dbl[])
              }
              frame 1, Default {
                # "Don't read: pass previous"
                n96 = Array Subset(array=w470, index=0, length=6) -> (w471:dbl[])
                n97 = Array Subset(array=w470, index=6, length=6) -> (w467:dbl[])
              }
            }
            "Voltages" <- w351
            "Vmon (V)" <- w351
            "IMon (uA)" <- w350
            n98 = Build Array("Apply Voltage", "Set to zero", "Kill voltage") -> (w314:bool[])
            n99 = Search 1D Array(1D array=w314, element=TRUE) -> (index of element=w334:i32)  [unwired: 1 in]
            n100 = case shown="0" w334 {
              tunnel: w333 -> [w374 w404 w434 w446]
              tunnel: w332 -> [w360 w393 w423 w448]
              tunnel: w331 -> [w370 w401 w431 w449]
              tunnel: w330 -> [w358 w391 w421 w447]
              tunnel: [w371 w402 w432 w446] -> w324
              tunnel: [w370 w401 w431 w449] -> w329
              tunnel: [w357 w390 w420 w448] -> w326
              tunnel: [w358 w391 w421 w447] -> w327
              tunnel: "VSet (V)" -> [w368 _ w429 _]
              tunnel: "VMax (V)" -> [w367 w399 _ _]
              tunnel: "IMax (uA)" -> [w366 w398 w428 _]
              frame 0 {
                w359 = 4 ("length")
                w364 = 2 ("length")
                w365 = 4 ("length")
                # "CAEN 2: Top gate, Bottom gate"
                # "CAEN 1 set values:\nPMT1&2, Anode, Cathode"
                # "Apply voltage"
                n101 = Array Subset(array=w368, length=w365) -> (w373:dbl[])  [unwired: 1 in]
                n102 = Array Subset(array=w367, length=w365) -> (w372:dbl[])  [unwired: 1 in]
                n103 = Array Subset(array=w366, length=w365) -> (w369:dbl[])  [unwired: 1 in]
                n104 = Array Subset(array=w366, index=w359, length=w364) -> (w361:dbl[])
                n105 = Array Subset(array=w368, index=w359, length=w364) -> (w363:dbl[])
                n106 = Array Subset(array=w367, index=w359, length=w364) -> (w362:dbl[])
                n107 = for {
                  tunnel: w370 -> [w384]
                  tunnel: w374 -> [w383]
                  tunnel: w373 -> [w380] mode=indexing
                  tunnel: w372 -> [w378] mode=indexing
                  tunnel: w369 -> [w377] mode=indexing
                  tunnel: [w376] -> w371
                  i -> [w385]
                  n108 = call "SET_SUPPLY_CHANNEL.vi"("VISA resource name"=w384, "Voltage Level (0.0 V)"=w380, "Enable (OFF)"=TRUE, "Board address"=u8 0, "NChannels"=u8 4, "Channel (0)"=w385, "error in (no error)"=w383, "Voltage Max (0.0 V)"=w378, "Current Limit (0.00 uA)"=w377) -> ("error out"=w376:errorcluster)  [unwired: 6 in]
                }
                n109 = for {
                  tunnel: w358 -> [_]
                  tunnel: w360 -> [w375]
                  tunnel: w363 -> [_] mode=indexing
                  tunnel: w362 -> [_] mode=indexing
                  tunnel: w361 -> [_] mode=indexing
                  tunnel: [w375] -> w357
                  # "CAEN 2 SET SUPPLY"
                }
              }
              frame 1 {
                w386 = 0 ("length")
                w388 = 0 ("length")
                w392 = 4 ("length")
                w396 = 2 ("length")
                w397 = 4 ("length")
                # "CAEN 2: Top gate, Bottom gate"
                # "CAEN 1 values:\nPMT1&2, Anode, Cathode"
                # "Set V to zero"
                n110 = Build Array(w388, w388, w388, w388) -> (w389:i32[])
                n111 = Array Subset(array=w398, length=w397) -> (w400:dbl[])  [unwired: 1 in]
                n112 = Array Subset(array=w399, length=w397) -> (w403:dbl[])  [unwired: 1 in]
                n113 = Build Array(w386, w386) -> (w387:i32[])
                n114 = Array Subset(array=w398, index=w392, length=w396) -> (w394:dbl[])
                n115 = Array Subset(array=w399, index=w392, length=w396) -> (w395:dbl[])
                n116 = for {
                  tunnel: w401 -> [w414]
                  tunnel: w404 -> [w413]
                  tunnel: w389 -> [w410] mode=indexing
                  tunnel: w403 -> [w408] mode=indexing
                  tunnel: w400 -> [w407] mode=indexing
                  tunnel: [w406] -> w402
                  i -> [w415]
                  n117 = call "SET_SUPPLY_CHANNEL.vi"("VISA resource name"=w414, "Voltage Level (0.0 V)"=w410, "Enable (OFF)"=TRUE, "Board address"=u8 0, "NChannels"=u8 4, "Channel (0)"=w415, "error in (no error)"=w413, "Voltage Max (0.0 V)"=w408, "Current Limit (0.00 uA)"=w407) -> ("error out"=w406:errorcluster)  [unwired: 6 in]
                }
                n118 = for {
                  tunnel: w391 -> [_]
                  tunnel: w393 -> [w405]
                  tunnel: w387 -> [_] mode=indexing
                  tunnel: w395 -> [_] mode=indexing
                  tunnel: w394 -> [_] mode=indexing
                  tunnel: [w405] -> w390
                  # "CAEN 2 SET SUPPLY CH 2"
                }
              }
              frame 2 {
                w417 = 0 ("length")
                w419 = 0 ("length")
                w422 = 4 ("length")
                w426 = 2 ("length")
                w427 = 4 ("length")
                # "CAEN 2: Top gate, Bottom gate"
                # "CAEN 1 values:\nPMT1&2, Anode, Cathode"
                # "Set VMax to zero, \"Kill\""
                n119 = Array Subset(array=w428, length=w427) -> (w430:dbl[])  [unwired: 1 in]
                n120 = Array Subset(array=w429, length=w427) -> (w433:dbl[])  [unwired: 1 in]
                n121 = Build Array(w419, w419, w419, w419) -> (w418:i32[])
                n122 = Array Subset(array=w428, index=w422, length=w426) -> (w424:dbl[])
                n123 = Array Subset(array=w429, index=w422, length=w426) -> (w425:dbl[])
                n124 = Build Array(w417, w417) -> (w416:i32[])
                n125 = for {
                  tunnel: w431 -> [w444]
                  tunnel: w434 -> [w443]
                  tunnel: w433 -> [w440] mode=indexing
                  tunnel: w418 -> [w438] mode=indexing
                  tunnel: w430 -> [w437] mode=indexing
                  tunnel: [w436] -> w432
                  i -> [w445]
                  n126 = call "SET_SUPPLY_CHANNEL.vi"("VISA resource name"=w444, "Voltage Level (0.0 V)"=w440, "Enable (OFF)"=TRUE, "Board address"=u8 0, "NChannels"=u8 4, "Channel (0)"=w445, "error in (no error)"=w443, "Voltage Max (0.0 V)"=w438, "Current Limit (0.00 uA)"=w437) -> ("error out"=w436:errorcluster)  [unwired: 6 in]
                }
                n127 = for {
                  tunnel: w421 -> [_]
                  tunnel: w423 -> [w435]
                  tunnel: w425 -> [_] mode=indexing
                  tunnel: w416 -> [_] mode=indexing
                  tunnel: w424 -> [_] mode=indexing
                  tunnel: [w435] -> w420
                  # "CAEN 2 SET SUPPLY CH 2"
                }
              }
              frame 3, Default {
                # "\"Executes\" if none of the three buttons have been clicked"
                # "Do nothing"
              }
            }
            n128 = Index Array(array=w335, index #1=0 ("index"), index #2=1 ("index"), index #3=2 ("index"), index #4=3 ("index"), index #5=4 ("index"), index #6=5 ("index")) -> (element #1=→"PMT 1":dbl, element #2=→"PMT 2":dbl, element #3=→"Anode":dbl, element #4=→"Cathode":dbl, element #5=→"Top gate":dbl, element #6=→"Bottom gate":dbl)
            n129 = Bundle("VISA resource name out"=w329, "error out"=w324) -> (w328:T3)  [unwired: 1 in]
            n130 = Bundle("VISA resource name out"=w327, "error out"=w326) -> (w325:T3)  [unwired: 1 in]
          }
          frame #3 {
            # "Descr."
            # "Reset anode"
            n131 = Search 1D Array(1D array=w486, element=TRUE) -> (index of element=w477:i32)  [unwired: 1 in]
            n132 = Not Equal?(x=w477, y=-1) -> (x != y?=w482:bool)
            n133 = case shown="True" "Reset anode" {
              tunnel: w485 -> [_ w509]
              tunnel: w484 -> [_ w521]
              tunnel: w483 -> [_ w490]
              tunnel: w482 -> [_ w511]
              tunnel: [w487 w491] -> w479
              frame False {
                # "Anode Reset Routine inactive:\nkeep timers up to date so activating\nroutine will correctly initiate the timers."
                n134 = Get Date/Time In Seconds() -> (seconds since 1Jan1904=w489:timestamp)
                n135 = To Double Precision Float(number=w489) -> (double precision float=w488:dbl)
                n136 = Build Array(w488, w488) -> (w487:dbl[])
              }
              frame True {
                # "0: 1st timer reset, 1: both timers reset, else: do nothing"
                # "Timers"
                # "0: Set to zero, 1: set to value, else: do nothing"
                # "Resetting the timers"
                # "Change Anode Voltage"
                # "Anode Imax"
                # "Anode Vmax"
                # "Anode Vset"
                # "Current time > total routine time?"
                # "Current time > target autokill time?"
                n137 = Get Date/Time In Seconds() -> (seconds since 1Jan1904=w523:timestamp)
                n138 = To Double Precision Float(number=w523) -> (double precision float=w504:dbl)
                n139 = Index Array(array=w509, index #1=0 ("index"), index #2=1 ("index")) -> (element #1=w503:dbl, element #2=w505:dbl)
                n140 = Multiply(x="Kill every Y minutes", y=60) -> (x*y=w501:i32)
                n141 = Unbundle(w521) -> ("VISA resource name out"=w520:refnum<visa-resource-name>, "error out"=w519:errorcluster)
                n142 = Subtract(x=w504, y=w503) -> (x-y=w502:dbl)
                n143 = Subtract(x=w504, y=w505) -> (x-y=w493:dbl)
                n144 = Add(x=w501, y="Keep off for X seconds") -> (x+y=w492:i32)
                n145 = Greater?(x=w502, y=w501) -> (0:w495:bool)
                "Killed" <- w495
                n146 = Greater?(x=w493, y=w492) -> (0:w496:bool)
                "Restarted" <- w496
                n147 = Or(x=w496, y=w511) -> (x .or. y?=w499:bool)
                n148 = Build Array(w495, w496) -> (w513:bool[])
                n149 = Build Array(w495, w499) -> (w500:bool[])
                n150 = Index Array(array=w490, index #1=2 ("index"), index #2=8 ("index"), index #3=14 ("index")) -> (element #1=w516:dbl, element #2=w514:dbl, element #3=w515:dbl)
                n151 = Search 1D Array(1D array=w513, element=TRUE) -> (index of element=w512:i32)  [unwired: 1 in]
                n152 = Search 1D Array(1D array=w500, element=TRUE) -> (index of element=w497:i32)  [unwired: 1 in]
                n153 = case shown="0" w512 {
                  tunnel: w516 -> [_ w548 _]
                  tunnel: w514 -> [w536 w547 _]
                  tunnel: w515 -> [w538 w546 _]
                  tunnel: w520 -> [w544 w551 _]
                  tunnel: w519 -> [w543 w550 _]
                  frame 0 {
                    # "Anode Vset to zero"
                    n154 = call "SET_SUPPLY_CHANNEL.vi"("VISA resource name"=w544, "Voltage Level (0.0 V)"=0.0, "Enable (OFF)"=TRUE, "Board address"=u8 0, "NChannels"=u8 4, "Channel (0)"=u8 2, "error in (no error)"=w543, "Voltage Max (0.0 V)"=w536, "Current Limit (0.00 uA)"=w538) -> ("error out"=w537:errorcluster)  [unwired: 6 in]
                    n155 = call <vilib>:"Simple Error Handler.vi"("error in (no error)"=w537) -> ()  [unwired: 4 in, 5 out]
                  }
                  frame 1 {
                    # "Anode Vset applied"
                    n156 = call "SET_SUPPLY_CHANNEL.vi"("VISA resource name"=w551, "Voltage Level (0.0 V)"=w548, "Enable (OFF)"=TRUE, "Board address"=u8 0, "NChannels"=u8 4, "Channel (0)"=u8 2, "error in (no error)"=w550, "Voltage Max (0.0 V)"=w547, "Current Limit (0.00 uA)"=w546) -> ("error out"=w545:errorcluster)  [unwired: 6 in]
                    n157 = call <vilib>:"Simple Error Handler.vi"("error in (no error)"=w545) -> ()  [unwired: 4 in, 5 out]
                  }
                  frame 2, Default {
                    # "Do nothing"
                  }
                }
                n158 = case shown="0" w497 {
                  tunnel: [w525 w531 w534] -> w491
                  tunnel: w509 -> [w529 _ w534]
                  frame 0 {
                    # "Only reset 1st timer, so it\ndoesn't stay True and lock-\nout 2nd check"
                    n159 = Get Date/Time In Seconds() -> (seconds since 1Jan1904=w528:timestamp)
                    n160 = Index Array(array=w529, index=1) -> (element=w526:dbl)
                    n161 = To Double Precision Float(number=w528) -> (double precision float=w527:dbl)
                    n162 = Build Array(w527, w526) -> (w525:dbl[])
                  }
                  frame 1 {
                    # "Reset timers if any button is pressed,\nor if the anode ramps up again"
                    n163 = Get Date/Time In Seconds() -> (seconds since 1Jan1904=w533:timestamp)
                    n164 = To Double Precision Float(number=w533) -> (double precision float=w532:dbl)
                    n165 = Build Array(w532, w532) -> (w531:dbl[])
                  }
                  frame 2, Default {
                    # "Time difference grows \nlarger for now"
                  }
                }
              }
            }
            "Anode times" <- w479
            n166 = To Time Stamp(1:w479) -> (0:→"Anode times 2":timestamp[])
            "?" <- "Reset anode"
          }
          frame #4 {
            # "<- for testing"
            # "Descr."
            # "Moving averages"
            # "Plots heater power vs. t"
            # "Historic graphs: Phase, Pressure, Flow, Heater, Temperature"
            # "Plots flow vs. t"
            # "Plots three pressures vs. t in one graph"
            # "Non-historic Temperature + Det. Pressure"
            # "Det., Low, High, Flow, Heater\nentire columns"
            # "Latest readings (NI, LS)"
            # "Single Temp.'s"
            # "Single Temp.'s"
            # "Updated TOBA"
            # "Descr."
            # "Latest Detector Pressure"
            # "Plots individual lists of Temp. vs. t"
            # "Plots and moving averages"
            n167 = Build Array (concatenate)(w598, w591) -> (w555:dbl[][])
            "TOBA appended" <- w555
            n168 = case shown="\"Average 15 to 20\", Default" "Temp. Channel selector" {
              tunnel: w591 -> [w661 w663 w666 w669 w672 w675 w678 w681 w688]
              tunnel: [w659 w662 w665 w668 w671 w674 w677 w680 w683] -> w601
              frame "Channel 15" {
                n169 = Index Array(array=w661, index=14) -> (element=w659:dbl)
              }
              frame "Channel 16" {
                n170 = Index Array(array=w663, index=15) -> (element=w662:dbl)
              }
              frame "Channel 17" {
                n171 = Index Array(array=w666, index=16) -> (element=w665:dbl)
              }
              frame "Channel 18" {
                n172 = Index Array(array=w669, index=17) -> (element=w668:dbl)
              }
              frame "Channel 19" {
                n173 = Index Array(array=w672, index=18) -> (element=w671:dbl)
              }
              frame "Channel 20" {
                n174 = Index Array(array=w675, index=19) -> (element=w674:dbl)
              }
              frame "Channel A" {
                n175 = Index Array(array=w678, index=20) -> (element=w677:dbl)
              }
              frame "Channel B" {
                n176 = Index Array(array=w681, index=21) -> (element=w680:dbl)
              }
              frame "Average 15 to 20", Default {
                w684 = 6 ("length")
                n177 = Array Subset(array=w688, index=14, length=w684) -> (w686:dbl[])
                n178 = Add Array Elements(numeric array=w686) -> (sum=w685:dbl)
                n179 = Divide(x=w685, y=w684) -> (x/y=w683:dbl)
              }
            }
            n180 = case shown="\"Channel 17\", Default" "Temperature Channel selector" {
              tunnel: w555 -> [w606 w609 w612 w615 w618 w621 w624 w627]
              tunnel: [w605 w608 w611 w614 w617 w620 w623 w626] -> w588
              frame "Channel 15" {
                n181 = Index Array(array=w606, index (col)=14) -> (element=w605:dbl[])  [unwired: 1 in]
              }
              frame "Channel 16" {
                n182 = Index Array(array=w609, index (col)=15) -> (element=w608:dbl[])  [unwired: 1 in]
              }
              frame "Channel 17", Default {
                n183 = Index Array(array=w612, index (col)=16) -> (element=w611:dbl[])  [unwired: 1 in]
              }
              frame "Channel 18" {
                n184 = Index Array(array=w615, index (col)=17) -> (element=w614:dbl[])  [unwired: 1 in]
              }
              frame "Channel 19" {
                n185 = Index Array(array=w618, index (col)=18) -> (element=w617:dbl[])  [unwired: 1 in]
              }
              frame "Channel 20" {
                n186 = Index Array(array=w621, index (col)=19) -> (element=w620:dbl[])  [unwired: 1 in]
              }
              frame "Channel A" {
                n187 = Index Array(array=w624, index (col)=20) -> (element=w623:dbl[])  [unwired: 1 in]
              }
              frame "Channel B" {
                n188 = Index Array(array=w627, index (col)=21) -> (element=w626:dbl[])  [unwired: 1 in]
              }
            }
            n189 = for {
              N: 22 -> [_]
              tunnel: w571 -> [w693]
              tunnel: [w692] -> w603 mode=indexing
              tunnel: w555 -> [w691]
              i -> [w690]
              n190 = Index Array(array=w691, index (col)=w690) -> (element=w689:dbl[])  [unwired: 1 in]
              n191 = Bundle(w693, w689) -> (w692:cluster{timestamp[], dbl[]})  [unwired: 1 in]
            }
            "Temperature" <- w603
            n192 = Index Array(array=w555, index (col) #1=23 ("disabled index (col)"), index (col) #2=24 ("index (col)"), index (col) #3=25 ("index (col)"), index (col) #4=26 ("index (col)"), index (col) #5=22 ("index (col)")) -> (element #1=w570:dbl[], element #2=w583:dbl[], element #3=w582:dbl[], element #4=w563:dbl[], element #5=w573:dbl[])  [unwired: 5 in]
            n193 = Index Array(array=w591, index=23) -> (element=w592:dbl)
            n194 = Bundle(w588, w570) -> (w587:cluster{dbl[], dbl[]})  [unwired: 1 in]
            n195 = Bundle("Heater 1 (%)"=w601, "Heater 1 (%)"=w592) -> (w600:cluster{"Heater 1 (%)":dbl, "Heater 1 (%)":dbl})  [unwired: 1 in]
            n196 = Bundle(w571, w570) -> (w581:cluster{timestamp[], dbl[]})  [unwired: 1 in]
            n197 = Bundle(w571, w583) -> (w580:cluster{timestamp[], dbl[]})  [unwired: 1 in]
            n198 = Bundle(w571, w582) -> (w579:cluster{timestamp[], dbl[]})  [unwired: 1 in]
            n199 = Bundle(w571, w563) -> (w576:cluster{timestamp[], dbl[]})  [unwired: 1 in]
            n200 = Bundle(w571, w573) -> (w572:cluster{timestamp[], dbl[]})  [unwired: 1 in]
            n201 = Build Array(w600) -> (→"Phase Diagram":T5)
            n202 = Build Array(w587) -> (→"Historical Large Phase Diagram":cluster{dbl[], dbl[]}[])
            n203 = Build Array(w581, w580, w579) -> (→"Pressure":cluster{timestamp[], dbl[]}[])
            n204 = Build Array(w576) -> (→"Flow (SLPM)":cluster{timestamp[], dbl[]}[])
            n205 = Build Array(w572) -> (→"Heater power (%)" →"Heater power (%) 2":cluster{timestamp[], dbl[]}[])
            n206 = case shown="\"Average 15 to 20\", Default" "Temperature Channel selector" {
              tunnel: w591 -> [w631 w633 w636 w639 w642 w645 w648 w651 w658]
              tunnel: [w629 w632 w635 w638 w641 w644 w647 w650 w653] -> w596
              frame "Channel 15" {
                n207 = Index Array(array=w631, index=14) -> (element=w629:dbl)
              }
              frame "Channel 16" {
                n208 = Index Array(array=w633, index=15) -> (element=w632:dbl)
              }
              frame "Channel 17" {
                n209 = Index Array(array=w636, index=16) -> (element=w635:dbl)
              }
              frame "Channel 18" {
                n210 = Index Array(array=w639, index=17) -> (element=w638:dbl)
              }
              frame "Channel 19" {
                n211 = Index Array(array=w642, index=18) -> (element=w641:dbl)
              }
              frame "Channel 20" {
                n212 = Index Array(array=w645, index=19) -> (element=w644:dbl)
              }
              frame "Channel A" {
                n213 = Index Array(array=w648, index=20) -> (element=w647:dbl)
              }
              frame "Channel B" {
                n214 = Index Array(array=w651, index=21) -> (element=w650:dbl)
              }
              frame "Average 15 to 20", Default {
                w654 = 6 ("length")
                n215 = Array Subset(array=w658, index=14, length=w654) -> (w656:dbl[])
                n216 = Add Array Elements(numeric array=w656) -> (sum=w655:dbl)
                n217 = Divide(x=w655, y=w654) -> (x/y=w653:dbl)
              }
            }
            n218 = Reverse 1D Array(array=w570) -> (reversed array=w569:dbl[])
            n219 = Reverse 1D Array(array=w563) -> (reversed array=w565:dbl[])
            n220 = Array Subset(array=w569, length="N samples") -> (w558:dbl[])  [unwired: 1 in]
            n221 = Array Subset(array=w565, length="N samples") -> (w560:dbl[])  [unwired: 1 in]
            n222 = Array Size(array=w560) -> (size(s)=w559:i32)
            n223 = Array Size(array=w558) -> (size(s)=w557:i32)
            n224 = Add Array Elements(numeric array=w560) -> (sum=w564:dbl)
            n225 = Add Array Elements(numeric array=w558) -> (sum=w568:dbl)
            n226 = Bundle("Heater 1 (%)"=w596, "Heater 1 (%)"=w592) -> (w597:cluster{"Heater 1 (%)":dbl, "Heater 1 (%)":dbl})  [unwired: 1 in]
            n227 = Divide(x=w564, y=w559) -> (x/y=→"Average Flow (SLPM)":dbl)
            n228 = Divide(x=w568, y=w557) -> (x/y=→"Moving average Det. P":dbl)
            n229 = Build Array(w597) -> (→"Large Phase Diagram":T5)
          }
          frame #5 {
            # "Temperatures (20),      NI Box;\nTemperatures (4),  Lakeshore;\nHeater Power,       Lakeshore;\nPressures (4),               NI Box;\nSetpoint,               Lakeshore;\nCurrent time (s)               ---   ;\nCycle time (s)                   ---   ;"
            # "Saving data"
            n230 = Get Date/Time In Seconds() -> (seconds since 1Jan1904=w707:timestamp)
            n231 = To Double Precision Float(number=w707) -> (double precision float=w706:dbl)
            n232 = Build Array (concatenate)(w709, w708, w706, w705, w704) -> (w703:dbl[])
            n233 = Get Date/Time String() -> (date string=w697:string)  [unwired: 3 in, 1 out]
            n234 = Build Path(base path=path "D:/Log_data/SC_LOG", name or relative path=w697) -> (appended path=w696:path)
            n235 = Format Date/Time String() -> (date/time string=w701:string)  [unwired: 3 in]
            n236 = Array To Spreadsheet String(array=w703, 3:"%.3f" ("format string")) -> (spreadsheet string=w699:string)  [unwired: 1 in]
            n237 = Concatenate Strings(w701, "\t", w699) -> (w695:string)
            n238 = call <vilib>:"Write Spreadsheet String.vi"("append to file? (new file:F)"=TRUE, "spreadsheet string"=w695, "file path (dialog if empty)"=w696) -> ()  [unwired: 7 in, 2 out]
          }
          frame #6 {
            # "Checking alarms"
            n239 = Unbundle By Name(w711) -> ("error out.status"=→"NI mod1 (P) status":bool)
            n240 = Unbundle By Name(w713) -> ("error out.status"=→"LakeShore status":bool)
            n241 = Unbundle By Name(w716) -> ("error out.status"=→"CAEN 1 status":bool)
            n242 = Unbundle By Name(w715) -> ("error out.status"=→"CAEN 2 status":bool)
          }
        }
        n243 = Decrement(x="Cycles to execute") -> (x-1=w131:dbl)
        n244 = Greater?(x=w143, y=w131) -> ()  [unwired: 1 out]
        n245 = Or(x=FALSE, y="stop") -> (x .or. y?=w146:bool)
      }
      "TOBA tester" <- w110
    }
    frame True {
    }
  }
  n246 = Array Size(array=w17) -> (size(s)=w20:i32)
  n247 = flat-sequence {
    tunnel: w4 -> [w730]
    frame #0 {
      w726 = u16 2 items=["1"=1, "2"=2] ("Heater Output (1:1)")
      w727 = u16 0 items=["Off", "Low (On)", "Medium", "High"] ("Range (0:Off)")
      # "Turn off heater, shutdown COM"
      # "Error Handling and Post-Processing (EHaPP)"
      n248 = Unbundle(w730) -> ("VISA resource name out"=w729:refnum<visa-resource-name>, "error out"=w728:errorcluster)
      n249 = call <instrlib>:"Configure Output Range and Manual Value.vi"("VISA resource name"=w729, "Heater Output (1:1)"=w726, "Range (0:Off)"=w727, "Manual Output (0.00 %)"=0.0, "error in (no error)"=w728) -> ("VISA resource name out"=w724:refnum<visa-resource-name>, "error out"=w723:errorcluster)  [unwired: 9 in]
      n250 = call <instrlib>:"Close.vi"("error in (no error)"=w723, "VISA resource name"=w724) -> ("error out"=w722:errorcluster)  [unwired: 9 in]
      n251 = call <vilib>:"Simple Error Handler.vi"("error in (no error)"=w722) -> ()  [unwired: 4 in, 5 out]
    }
  }
  n252 = Decrement(x=w20) -> (x-1=w19:i32)
  n253 = Index Array(array=w17, index=w19) -> (element=w18:timestamp)
  n254 = Index Array(array=w17, index=1) -> (element=w15:timestamp)
  n255 = To Double Precision Float(number=w18) -> (double precision float=w14:dbl)
  n256 = To Double Precision Float(number=w15) -> (double precision float=w13:dbl)
  n257 = Subtract(x=w14, y=w13) -> ()  [unwired: 1 out]
  "Started up?" <- w9
